vi "GenerateFilePaths.vi"(3 "error in (no error)":errorcluster, 5 "EpiWrapper in":refnum<class "EpiWrapper.lvclass">) -> (0 "error out":errorcluster, 1 "Errors":errorcluster[](array[cluster]), 2 "EpiWrapper out":refnum<class "EpiWrapper.lvclass">)   [LabVIEW 2012, in "EpiWrapper.lvclass"]
uses:
  EpiWrapper.lvclass
  EpiWrapper.lvclass/EpiWrapper.ctl
  Controls/Constants.vi
panel:
  out "appended path":path
  out "file or folder exists?":bool
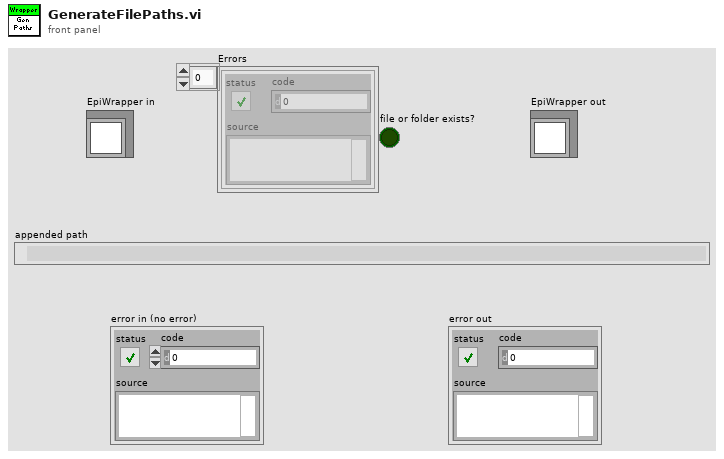
[diagram p1: front panel]
types:
  T1 = typedef "AppPaths.ctl" = cluster{"DataDir":T2, "OmniDriver":T2, "OmniDriverCommon":T2, "Configuration":T2, "WaferImage":T2}
  T2 = typedef "PathTraveler.ctl" = cluster{"Enum":T3, "FileName":string, "Exists?":bool, "Path":path}
  T3 = typedef "PathTypes.ctl" = enum16{"DataDir", "OmniDriver", "OmniDriver_Common", "Configuration", "WaferImage"}
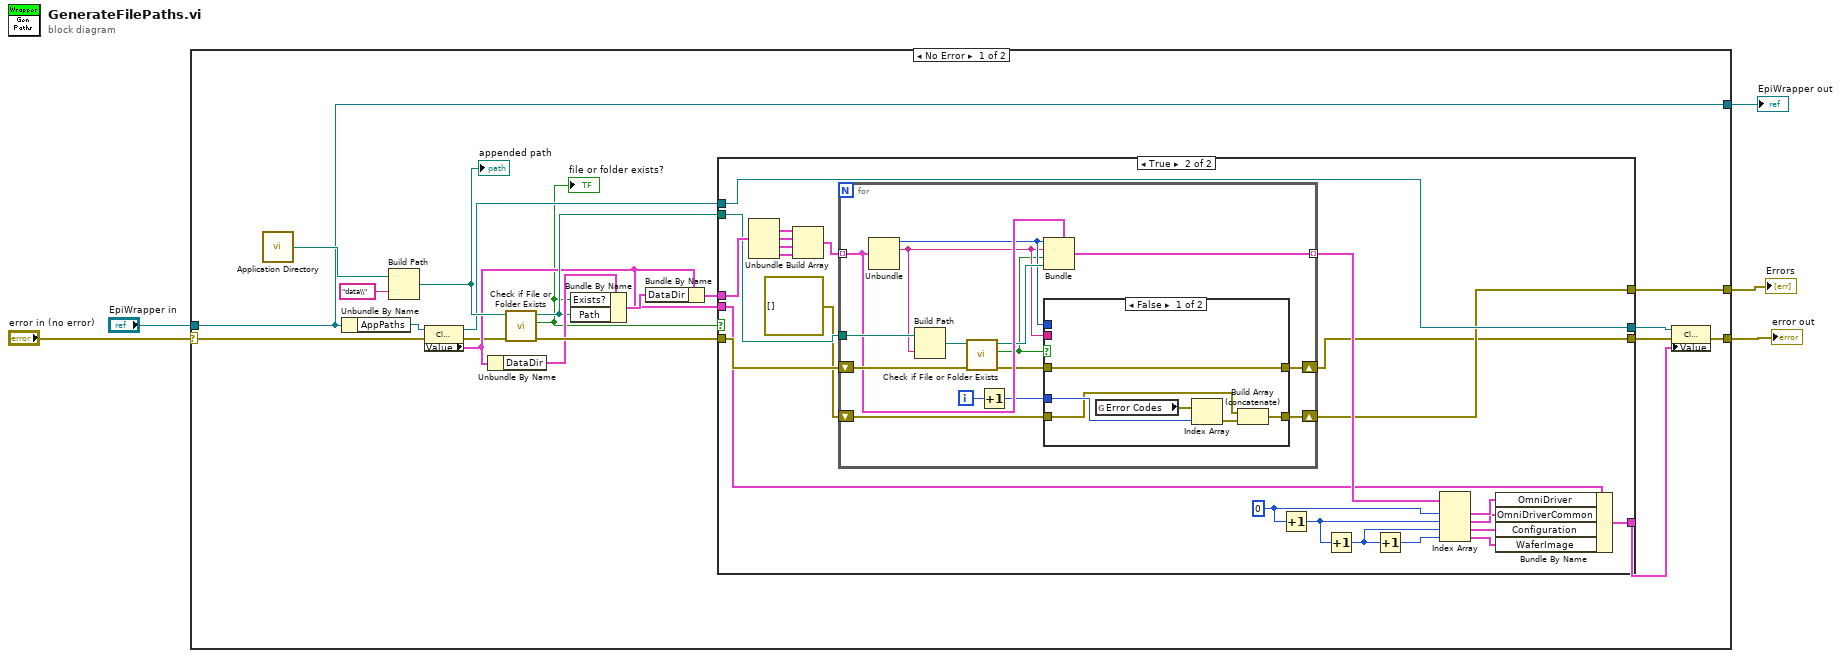
[diagram p0: block diagram]
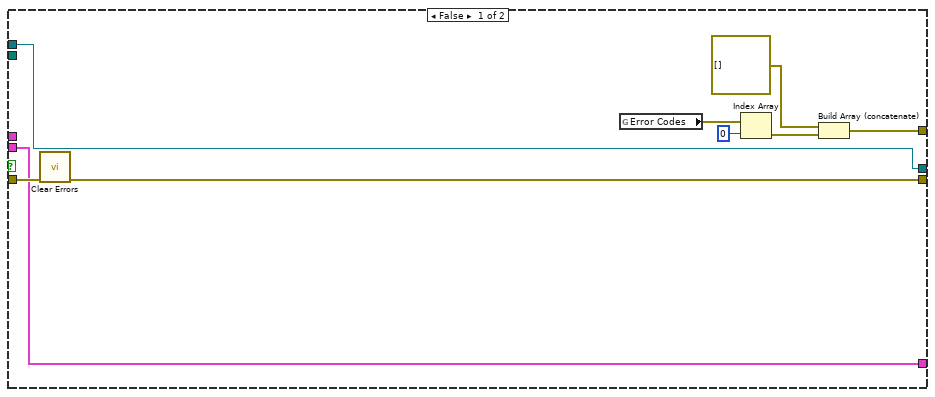
[diagram p2: hidden frame]
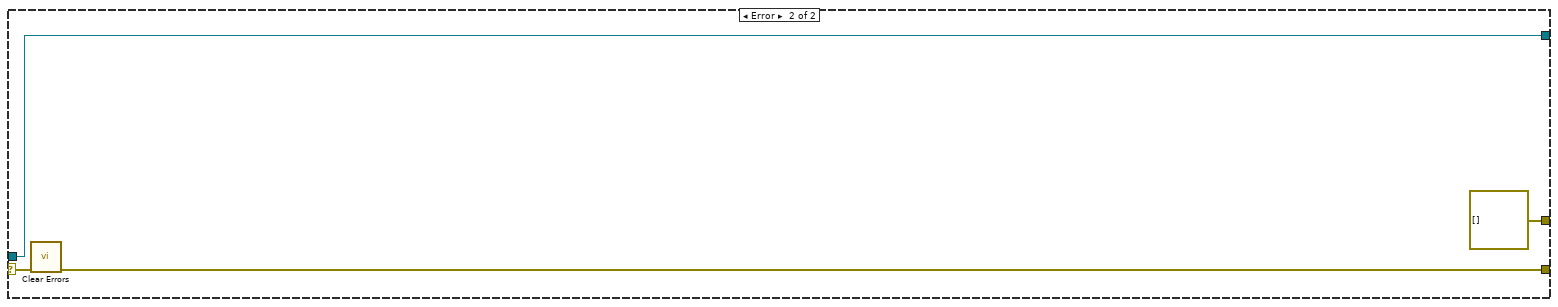
[diagram p4: hidden frame]
diagram:
  n1 = case shown="No Error" "error in (no error)" {
    selector: "error in (no error)" -> [w10 w83]
    tunnel: "EpiWrapper in" -> [w7 w84]
    tunnel: [w8 w82] -> w2
    tunnel: [w7 w84] -> w4
    tunnel: [w6 errorcluster[] []] -> w1
    frame No Error {
      n2 = call <vilib>:"Application Directory.vi"() -> ("Application Directory"=w25:path)
      n3 = Unbundle By Name(w7) -> ("AppPaths"=w9:refnum<vi>)
      n4 = Build Path(base path=w25, name or relative path="data\\") -> (appended path=w23:path)
      "appended path" <- w23
      n5 = property class="Clust (strict)"(reference=w9, error in=w10) -> (reference out=w15:refnum<vi>, error out=w16:errorcluster, "Value"=w17:T1)
      n6 = Unbundle By Name(w17) -> ("DataDir"=w21:T2)
      n7 = call <vilib>:"Check if File or Folder Exists.vi"("error in (no error)"=w16, "path"=w23) -> ("error out"=w22:errorcluster, "file or folder exists?"=w12:bool, "dup path"=w18:path)  [unwired: 7 in]
      "file or folder exists?" <- w12
      n8 = Bundle By Name(cluster=w21, "Exists?"=w12, "Path"=w18) -> (w20:T2)
      n9 = Bundle By Name(cluster=w17, "DataDir"=w20) -> (w19:T1)
      n10 = case shown="True" w12 {
        tunnel: w22 -> [w34 w50]
        tunnel: w19 -> [_ w57]
        tunnel: w18 -> [_ w51]
        tunnel: w17 -> [w33 w40]
        tunnel: w15 -> [w32 w39]
        tunnel: [w27 w35] -> w11
        tunnel: [w33 w38] -> w14
        tunnel: [w32 w39] -> w13
        tunnel: [w28 w36] -> w6
        frame False {
          n11 = call <vilib>:"Clear Errors.vi"("error in (no error)"=w34) -> ("error out"=w27:errorcluster)  [unwired: 6 in]
          n12 = global read "Constants.vi" "Error Codes"() -> (w31:errorcluster[])
          n13 = Index Array(array=w31, index=0) -> (element=w26:errorcluster)
          n14 = Build Array (concatenate)(errorcluster[] [], w26) -> (w28:errorcluster[])
        }
        frame True {
          w48 = 0 ("index")
          n15 = Unbundle(w57) -> ("OmniDriver"=w56:T2, "OmniDriverCommon"=w55:T2, "Configuration"=w54:T2, "WaferImage"=w53:T2)  [unwired: 1 out]
          n16 = Build Array(w56, w55, w54, w53) -> (w52:T2[])
          n17 = for {
            tunnel: w52 -> [w69] mode=indexing
            tunnel: w51 -> [w71]
            tunnel: [w68] -> w49 mode=indexing
            shift-right: [w61] -> w35
            shift-left: w50 -> [w70]
            shift-right: [w59] -> w36
            shift-left: errorcluster[] [] -> [w60]
            i -> [w63]
            n18 = Unbundle(w69) -> ("Enum"=w65:T3, "FileName"=w64:string)  [unwired: 2 out]
            n19 = Build Path(base path=w71, name or relative path=w64) -> (appended path=w72:path)
            n20 = call <vilib>:"Check if File or Folder Exists.vi"("error in (no error)"=w70, "path"=w72) -> ("error out"=w66:errorcluster, "file or folder exists?"=w62:bool, "dup path"=w67:path)  [unwired: 7 in]
            n21 = Increment(x=w63) -> (x+1=w58:i32)
            n22 = Bundle(cluster=w69, "Enum"=w65, "FileName"=w64, "Exists?"=w62, "Path"=w67) -> (w68:T2)
            n23 = case shown="False" w62 {
              tunnel: w66 -> [w78 w80]
              tunnel: w65 -> [_ _]
              tunnel: w64 -> [_ _]
              tunnel: [w78 w80] -> w61
              tunnel: w60 -> [w75 w79]
              tunnel: [w74 w79] -> w59
              tunnel: w58 -> [w76 _]
              frame False {
                n24 = global read "Constants.vi" "Error Codes"() -> (w77:errorcluster[])
                n25 = Index Array(array=w77, index=w76) -> (element=w73:errorcluster)
                n26 = Build Array (concatenate)(w75, w73) -> (w74:errorcluster[])
              }
              frame True {
              }
            }
          }
          n27 = Increment(x=w48) -> (x+1=w47:i32)
          n28 = Increment(x=w47) -> (x+1=w45:i32)
          n29 = Increment(x=w45) -> (x+1=w46:i32)
          n30 = Index Array(array=w49, index #1=w48, index #2=w47, index #3=w45, index #4=w46) -> (element #1=w44:T2, element #2=w43:T2, element #3=w42:T2, element #4=w41:T2)
          n31 = Bundle By Name(cluster=w40, "OmniDriver"=w44, "OmniDriverCommon"=w43, "Configuration"=w42, "WaferImage"=w41) -> (w38:T1)
        }
      }
      n32 = property class="Clust (strict)"(reference=w13, error in=w11, "Value"=w14) -> (error out=w8:errorcluster)  [unwired: 1 out]
    }
    frame Error {
      n33 = call <vilib>:"Clear Errors.vi"("error in (no error)"=w83) -> ("error out"=w82:errorcluster)  [unwired: 6 in]
    }
  }
  "EpiWrapper out" <- w4
  "error out" <- w2
  "Errors" <- w1
